vi "Register gRPC Methods.vi"(8 "error in (no error)":errorcluster, 11 "Template Server in":refnum<class "HVC8.lvclass">) -> (0 "error out":errorcluster, 3 "Template Server out":refnum<class "HVC8.lvclass">)   [LabVIEW 2019, in "HVC8.lvlib" / "HVC8.lvclass"]
uses:
  HVC8.lvclass
  typeDefs/Server Internal UEs.ctl
  typeDefs/Server Internal Message.ctl
  typeDefs/Server gRPC UEs.ctl
  gRPC lvSupport/Server API/typeDefs/gRPCId Cluster.ctl
  gRPC lvSupport/Server API/typeDefs/grpcId.ctl
  HVC8.lvclass/HVC8.ctl
  gRPC lvSupport/gprc-lvsupport.lvlib
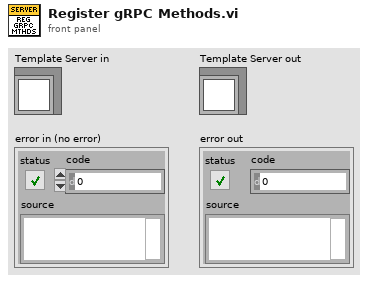
[diagram p1: front panel]
types:
  T1 = typedef "HVC8.lvlib/HVC8.lvclass/Server gRPC UEs.ctl" = cluster{"Invoke gRPC UE":refnum<user-event>, "Query gRPC UE":refnum<user-event>, "Register gRPC UE":refnum<user-event>, "OpenDISession gRPC UE":refnum<user-event>, "OpenDOSession gRPC UE":refnum<user-event>, "ReadDI gRPC UE":refnum<user-event>, "WriteDO gRPC UE":refnum<user-event>, "CloseDISession gRPC UE":refnum<user-event>, "CloseDOSession gRPC UE":refnum<user-event>}
  T2 = typedef "HVC8.lvlib/HVC8.lvclass/Server Internal UEs.ctl" = cluster{"Invoke Internal UE":refnum<user-event>, "Query Internal UE":refnum<user-event>, "Register Internal UE":refnum<user-event>, "OpenDISession Internal UE":refnum<user-event>, "OpenDOSession Internal UE":refnum<user-event>, "ReadDI Internal UE":refnum<user-event>, "WriteDO Internal UE":refnum<user-event>, "CloseDISession Internal UE":refnum<user-event>, "CloseDOSession Internal UE":refnum<user-event>}
  T3 = typedef "HVC8.lvlib/gprc-lvsupport.lvlib/grpcId.ctl" = u64
  T4 = typedef "HVC8.lvlib/HVC8.lvclass/Server Internal Message UE.ctl" = refnum<user-event>
  T5 = typedef "HVC8.lvlib/gprc-lvsupport.lvlib/gRPCId Cluster UE.ctl" = refnum<user-event>
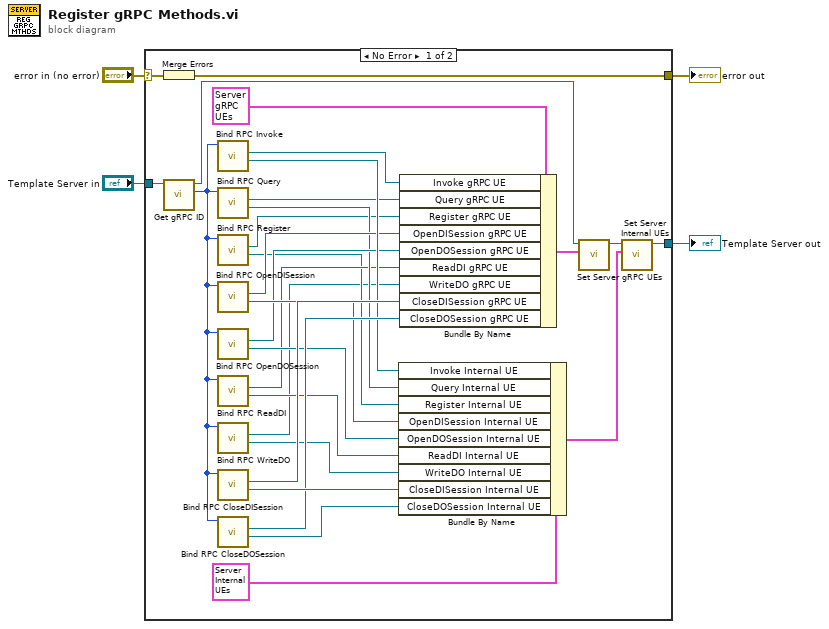
[diagram p0: block diagram]
diagram:
  n1 = case shown="No Error" "error in (no error)" {
    selector: "error in (no error)" -> [w24 w34]
    tunnel: "Template Server in" -> [w32 w35]
    tunnel: [w31 w34] -> w3
    tunnel: [w30 w35] -> w2
    frame No Error {
      n2 = Merge Errors(w24) -> (w31:errorcluster)
      n3 = call "Get gRPC ID.vi"("OOP Server in"=w32) -> ("gRPC ID"=w23:T3, "OOP Server out"=w33:refnum<class "HVC8.lvclass">)  [unwired: 9 in]
      n4 = call "Bind RPC Invoke.vi"("gRPCid server in"=w23) -> ("Invoke Internal UE"=w18:T4, "Invoke gRPC UE"=w17:T5)  [unwired: 7 in, 2 out]
      n5 = call "Bind RPC Query.vi"("gRPCid server in"=w23) -> ("Query Internal UE"=w12:T4, "Query gRPC UE"=w11:T5)  [unwired: 7 in, 2 out]
      n6 = call "Bind RPC Register.vi"("gRPCid server in"=w23) -> ("Register Internal UE"=w8:T4, "Register gRPC UE"=w7:T5)  [unwired: 7 in, 2 out]
      n7 = call "Bind RPC OpenDISession.vi"("gRPCid server in"=w23) -> ("OpenDISession Internal UE"=w16:T4, "OpenDISession gRPC UE"=w15:T5)  [unwired: 7 in, 2 out]
      n8 = call "Bind RPC OpenDOSession.vi"("gRPCid server in"=w23) -> ("OpenDOSession Internal UE"=w14:T4, "OpenDOSession gRPC UE"=w13:T5)  [unwired: 7 in, 2 out]
      n9 = call "Bind RPC ReadDI.vi"("gRPCid server in"=w23) -> ("ReadDI Internal UE"=w10:T4, "ReadDI gRPC UE"=w9:T5)  [unwired: 7 in, 2 out]
      n10 = call "Bind RPC WriteDO.vi"("gRPCid server in"=w23) -> ("WriteDO Internal UE"=w6:T4, "WriteDO gRPC UE"=w5:T5)  [unwired: 7 in, 2 out]
      n11 = call "Bind RPC CloseDISession.vi"("gRPCid server in"=w23) -> ("CloseDISession Internal UE"=w22:T4, "CloseDISession gRPC UE"=w21:T5)  [unwired: 7 in, 2 out]
      n12 = call "Bind RPC CloseDOSession.vi"("gRPCid server in"=w23) -> ("CloseDOSession Internal UE"=w20:T4, "CloseDOSession gRPC UE"=w19:T5)  [unwired: 7 in, 2 out]
      n13 = Bundle By Name ("Bundle Internal UEs")(cluster=T2 {"Invoke Internal UE"=refnum, "Query Internal UE"=refnum, "Register Internal UE"=refnum, "OpenDISession Internal UE"=refnum, "OpenDOSession Internal UE"=refnum, "ReadDI Internal UE"=refnum, "WriteDO Internal UE"=refnum, "CloseDISession Internal UE"=refnum, "CloseDOSession Internal UE"=refnum} ("Server Internal UEs"), "Invoke Internal UE"=w18, "Query Internal UE"=w12, "Register Internal UE"=w8, "OpenDISession Internal UE"=w16, "OpenDOSession Internal UE"=w14, "ReadDI Internal UE"=w10, "WriteDO Internal UE"=w6, "CloseDISession Internal UE"=w22, "CloseDOSession Internal UE"=w20) -> (w29:T2)
      n14 = Bundle By Name ("Bundle gRPC UEs")(cluster=T1 {"Invoke gRPC UE"=refnum, "Query gRPC UE"=refnum, "Register gRPC UE"=refnum, "OpenDISession gRPC UE"=refnum, "OpenDOSession gRPC UE"=refnum, "ReadDI gRPC UE"=refnum, "WriteDO gRPC UE"=refnum, "CloseDISession gRPC UE"=refnum, "CloseDOSession gRPC UE"=refnum} ("gRPC Server Method Events"), "Invoke gRPC UE"=w17, "Query gRPC UE"=w11, "Register gRPC UE"=w7, "OpenDISession gRPC UE"=w15, "OpenDOSession gRPC UE"=w13, "ReadDI gRPC UE"=w9, "WriteDO gRPC UE"=w5, "CloseDISession gRPC UE"=w21, "CloseDOSession gRPC UE"=w19) -> (w26:T1)
      n15 = call "Set Server gRPC UEs.vi"("Server gRPC UEs"=w26, "OOP Server in"=w33) -> ("OOP Server out"=w27:refnum<class "HVC8.lvclass">)  [unwired: 9 in]
      n16 = call "Set Server Internal UEs.vi"("Server Internal UEs"=w29, "OOP Server in"=w27) -> ("OOP Server out"=w30:refnum<class "HVC8.lvclass">)  [unwired: 9 in]
    }
    frame Error {
    }
  }
  "error out" <- w3
  "Template Server out" <- w2
